vi "Draw Selection.vi"(0 "Display State In":T1={"Nspeakers"=0, "actions"=[], "Wspeaker"=0, "hover"={"type"=enum."None", "index"=0}, "locked"=FALSE, "states"=[], "sel speak"=13, "selected"=refnum, "Events"={"Selection change"=refnum}}, 5 "Layout":T6) -> (4 "empty picture":picture, 8 "String":string)   [LabVIEW 2015, in "SAC Config.xctl"]
uses:
  SAC Config.xctl
  Layout.ctl
  Item.ctl
  State.vi
  Hover Data.ctl
  Hover Item.ctl
  Speaker State.ctl
  Events.ctl
  Selection changed.ctl
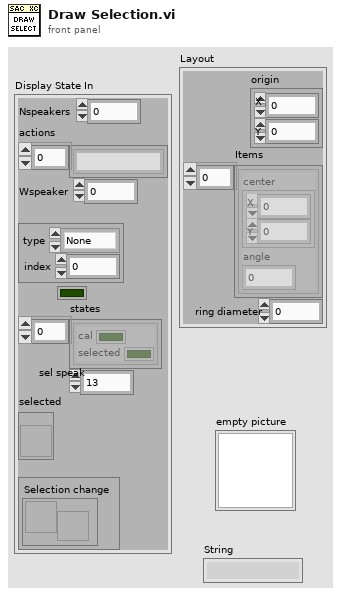
[diagram p1: front panel]
types:
  T1 = typedef "SAC Config.xctl/State.vi" = cluster{"Nspeakers":i32, "actions":string[], "Wspeaker":i32, "hover":T2, "locked":bool, "states":T4[], "sel speak":i32, "selected":refnum<vi>, "Events":T5}
  T2 = typedef "SAC Config.xctl/Hover Data.ctl" = cluster{"type":T3, "index":i32}
  T3 = typedef "SAC Config.xctl/Hover Item.ctl" = enum16{"None", "Speaker"}
  T4 = typedef "SAC Config.xctl/Speaker State.ctl" = cluster{"cal":bool, "selected":bool}
  T5 = typedef "SAC Config.xctl/Events.ctl" = cluster{"Selection change":refnum<user-event>}
  T6 = typedef "SAC Config.xctl/Layout.ctl" = cluster{"origin":cluster{"X":i32, "Y":i32}, "Items":T7[], "ring diameter":i32}
  T7 = typedef "SAC Config.xctl/Item.ctl" = cluster{"center":cluster{"X":i32, "Y":i32}, "angle":dbl}
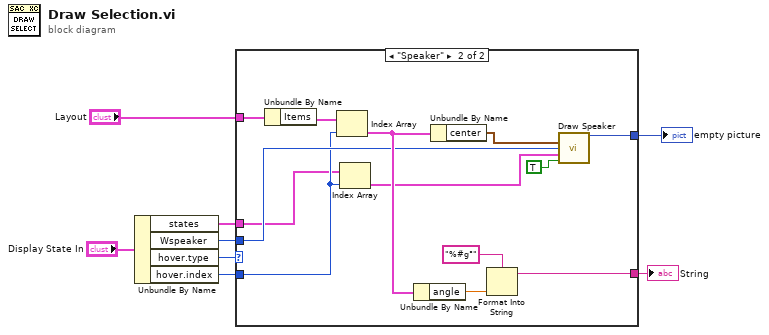
[diagram p0: block diagram]
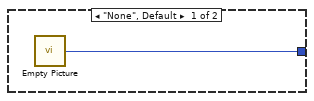
[diagram p2: hidden frame]
diagram:
  n1 = Unbundle By Name("Display State In") -> ("states"=w1:T4[], "Wspeaker"=w3:i32, "hover.type"=w5:T3, "hover.index"=w4:i32)
  n2 = case shown="\"Speaker\"" w5 {
    tunnel: "Layout" -> [_ w22]
    tunnel: [w9 w17] -> w8
    tunnel: w4 -> [_ w13]
    tunnel: w3 -> [_ w14]
    tunnel: [_ w18] -> w2
    tunnel: w1 -> [_ w12]
    frame "None", Default {
      n3 = call "Empty Picture"() -> ("empty picture"=w9:picture)
    }
    frame "Speaker" {
      n4 = Unbundle By Name(w22) -> ("Items"=w21:T7[])
      n5 = Index Array(array=w21, index=w13) -> (element=w16:T7)
      n6 = Index Array(array=w12, index=w13) -> (element=w11:T4)
      n7 = Unbundle By Name(w16) -> ("angle"=w20:dbl)
      n8 = Unbundle By Name(w16) -> ("center"=w15:cluster{"X":i32, "Y":i32})
      n9 = Format Into String(format string="%#g°", w20) -> (resulting string=w18:string)  [unwired: 2 in, 1 out]
      n10 = call "Draw Speaker.vi"("center"=w15, "width"=w14, "state"=w11, "active"=TRUE) -> ("picture out"=w17:picture)  [unwired: 11 in]
    }
  }
  "empty picture" <- w8
  "String" <- w2
